vi "PoseInDefenseArea.vi"(5 "theta":dbl, 7 "Recuo":dbl=130.0, 8 "geometry":T1, 9 "Ball":dbl[](array[numeric]), 10 "Field defense":dbl[](array[numeric]), 11 "Events.Ball out":bool) -> (3 "Array":dbl[](array[numeric]))   [LabVIEW 2016]
uses:
  Core/Field Size.ctl
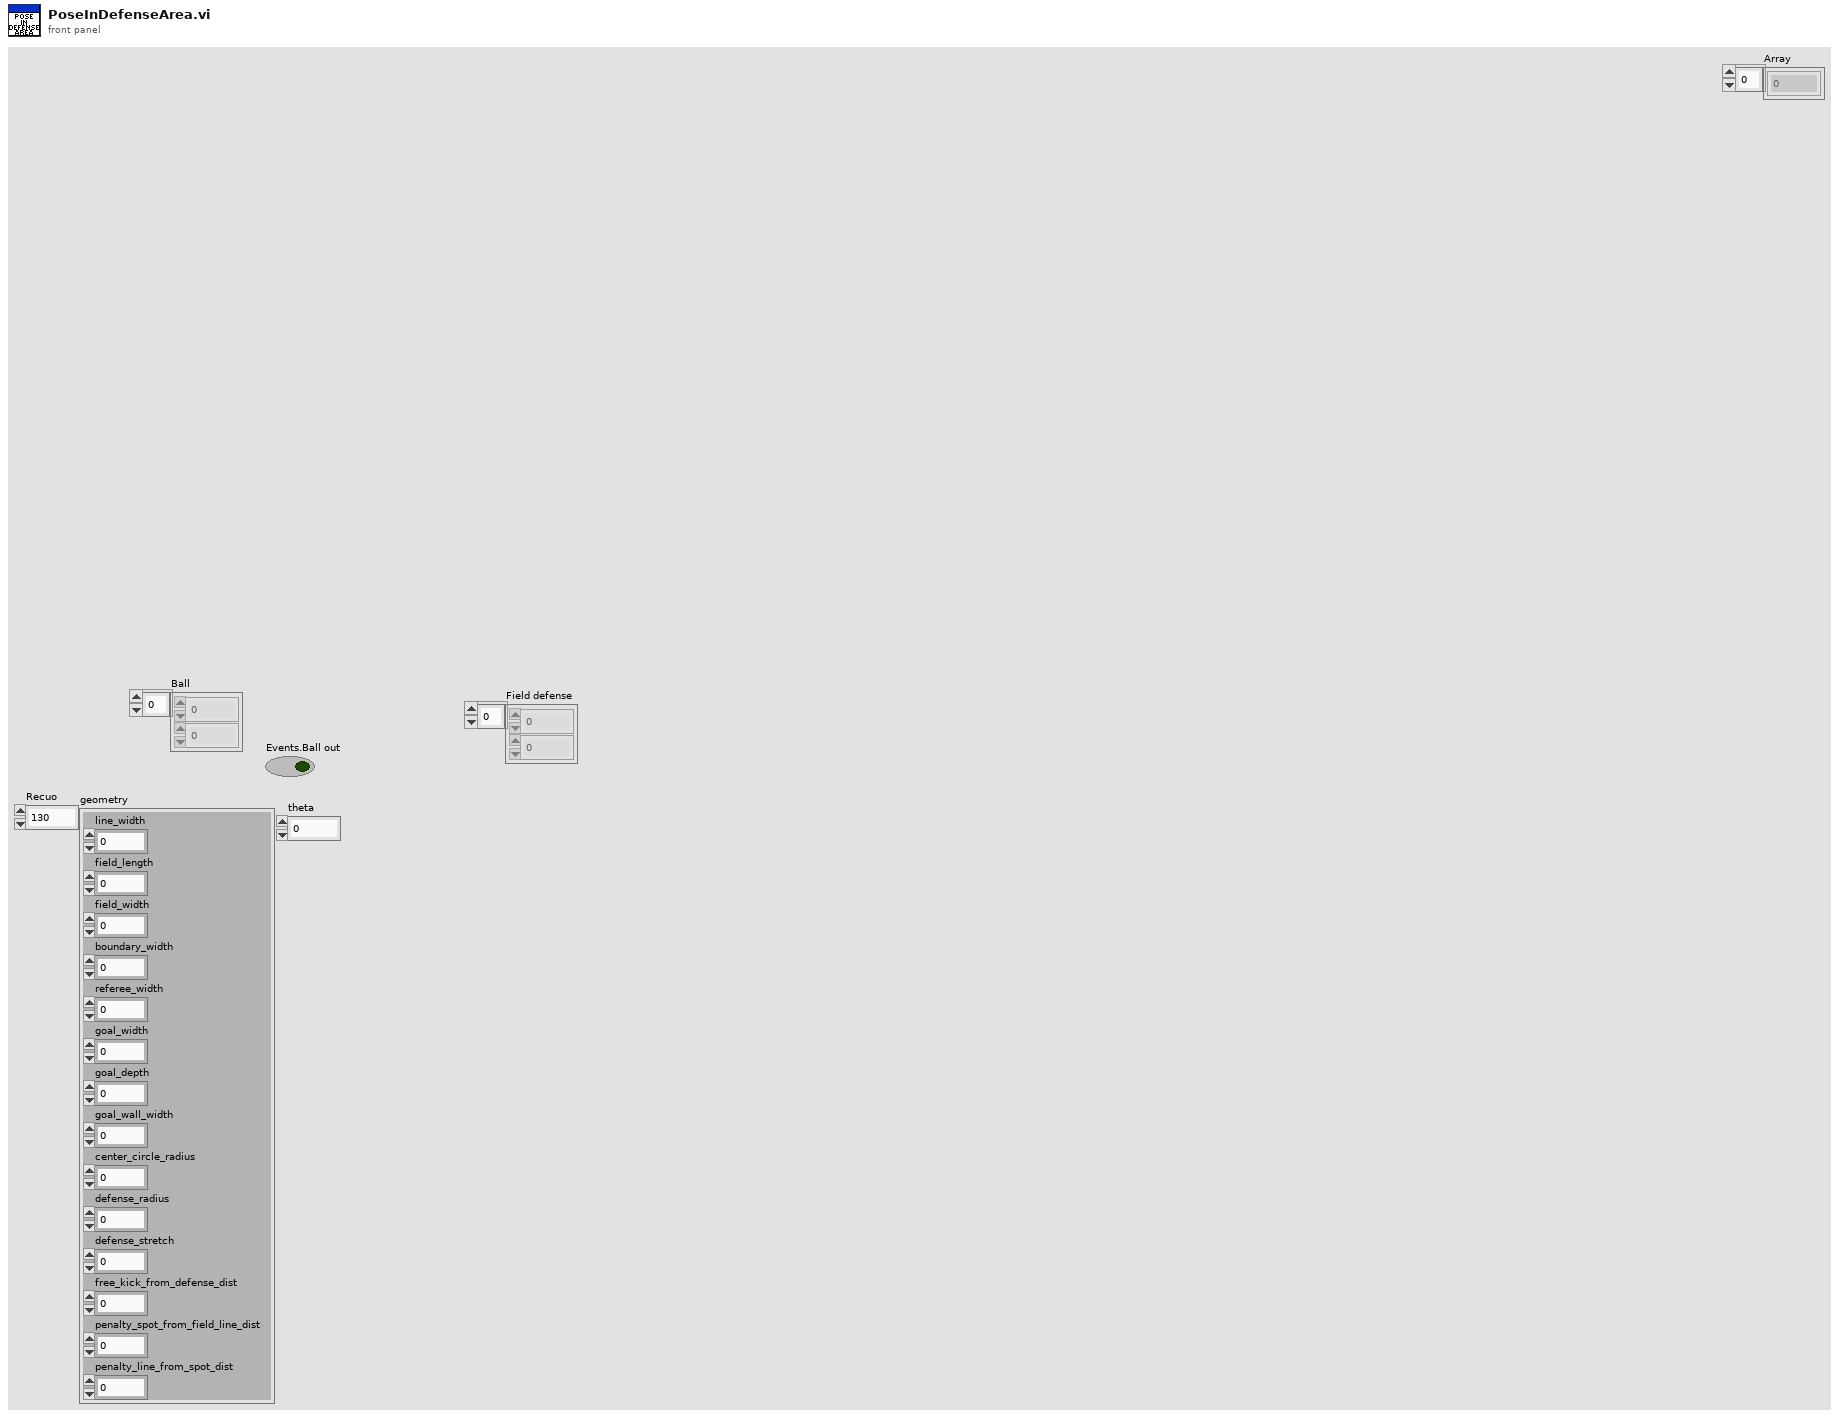
[diagram p1: front panel]
types:
  T1 = typedef "Field Size.ctl" = cluster{"line_width":u32, "field_length":u32, "field_width":u32, "boundary_width":u32, "referee_width":u32, "goal_width":u32, "goal_depth":u32, "goal_wall_width":u32, "center_circle_radius":u32, "defense_radius":u32, "defense_stretch":u32, "free_kick_from_defense_dist":u32, "penalty_spot_from_field_line_dist":u32, "penalty_line_from_spot_dist":u32}
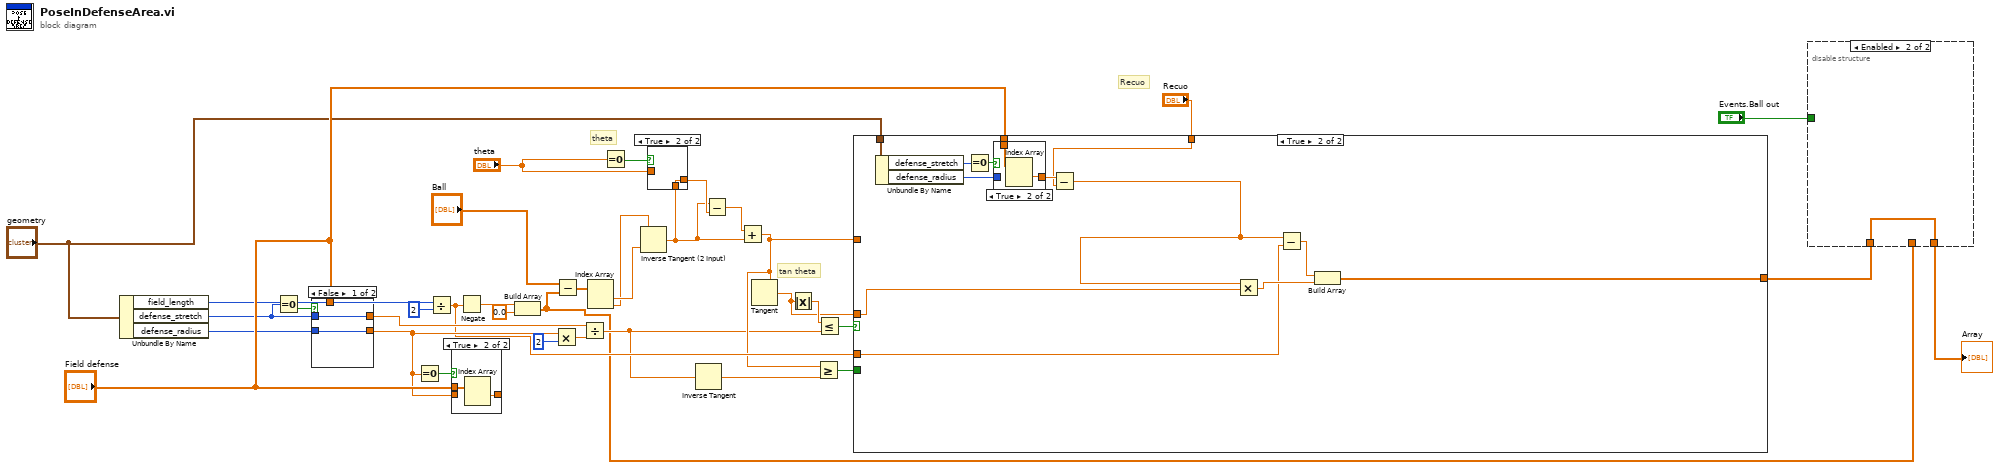
[diagram p0: block diagram]
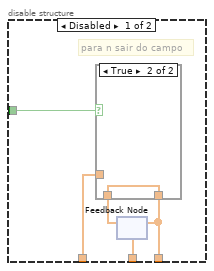
[diagram p2: hidden frame]
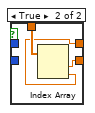
[diagram p5: hidden frame]
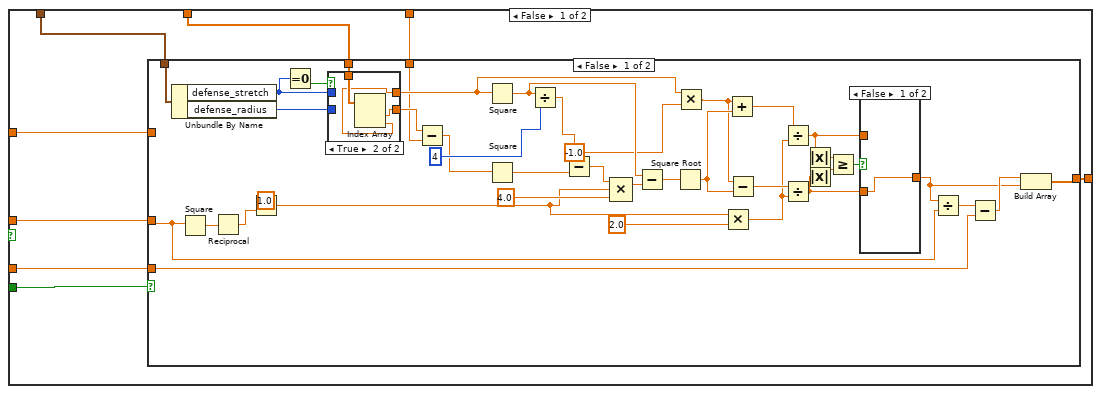
[diagram p6: hidden frame]
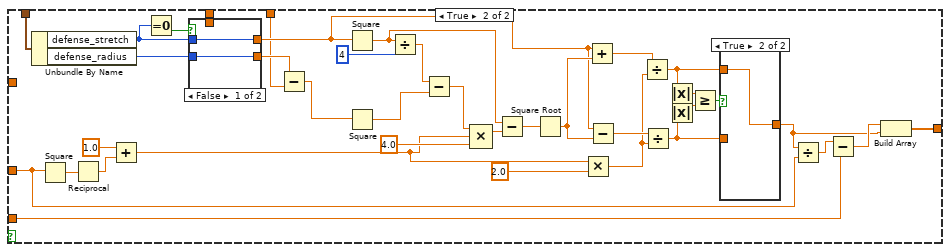
[diagram p9: hidden frame]
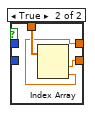
[diagram p10: hidden frame]
diagram:
  # "Recuo"
  # "tan theta"
  # "theta"
  n1 = Unbundle By Name("geometry") -> ("field_length"=w15:u32, "defense_stretch"=w32:u32, "defense_radius"=w31:u32)
  n2 = Equal To 0?(x=w32) -> (x = 0?=w30:bool)
  n3 = case shown="False" w30 {
    tunnel: w32 -> [w38 _]
    tunnel: [w38 w40] -> w34
    tunnel: [w37 w39] -> w33
    tunnel: w31 -> [w37 _]
    tunnel: "Field defense" -> [_ w41]
    frame False {
    }
    frame True {
      n4 = Index Array(array=w41) -> (element #1=w39:dbl, element #2=w40:dbl)  [unwired: 2 in]
    }
  }
  n5 = Equal To 0?(x=w33) -> (x = 0?=w14:bool)
  n6 = Divide(x=w15, y=u32 2) -> (x/y=w27:dbl)
  n7 = case shown="True" w14 {
    tunnel: [w42 w43] -> _
    tunnel: w33 -> [w42 _]
    tunnel: "Field defense" -> [_ w44]
    frame False {
    }
    frame True {
      n8 = Index Array(array=w44) -> (element #2=w43:dbl)  [unwired: 2 in, 1 out]
    }
  }
  n9 = Negate(x=w27) -> (-x=w17:dbl)
  n10 = Build Array(w17, 0.0 ("element")) -> (w2:dbl[])
  n11 = Multiply(x=w33, y=u32 2) -> (x*y=w21:dbl)
  n12 = Subtract(x="Ball", y=w2) -> (x-y=w19:dbl[])
  n13 = Divide(x=w34, y=w21) -> (x/y=w4:dbl)
  n14 = Index Array(array=w19) -> (element #1=w26:dbl, element #2=w25:dbl)  [unwired: 2 in]
  n15 = Equal To 0?(x="theta") -> (x = 0?=w8:bool)
  n16 = Inverse Tangent (2 Input)(1:w26, 2:w25) -> (0:w6:dbl)
  n17 = case shown="True" w8 {
    tunnel: [w45 w46] -> w9
    tunnel: "theta" -> [w45 _]
    tunnel: w6 -> [_ w46]
    frame False {
    }
    frame True {
    }
  }
  n18 = Inverse Tangent(1:w4) -> (0:w3:dbl)
  n19 = Subtract(x=w6, y=w9) -> (x-y=w10:dbl)
  n20 = Add(x=w10, y=w6) -> (x+y=w5:dbl)
  n21 = Tangent(1:w5) -> (0:w11:dbl)
  n22 = Absolute Value(x=w11) -> (abs(x)=w20:dbl)
  n23 = Greater Or Equal?(x=w5, y=w3) -> (x >= y?=w24:bool)
  n24 = Less Or Equal?(x=w20, y=w4) -> (x <= y?=w23:bool)
  n25 = case shown="True" w23 {
    tunnel: w5 -> [w49 _]
    tunnel: "geometry" -> [w53 w157]
    tunnel: [w51 w155] -> w28
    tunnel: w24 -> [w54 _]
    tunnel: w11 -> [w52 w152]
    tunnel: w27 -> [w50 w153]
    tunnel: "Field defense" -> [w48 w146]
    tunnel: "Recuo" -> [w47 w145]
    frame False {
      n26 = case shown="False" w54 {
        tunnel: w53 -> [w76 w137]
        tunnel: w52 -> [w75 w119]
        tunnel: [w74 w118] -> w51
        tunnel: w50 -> [w70 w116]
        tunnel: w49 -> [_ _]
        tunnel: w48 -> [w64 w107]
        tunnel: w47 -> [w55 w101]
        frame False {
          n27 = Unbundle By Name(w76) -> ("defense_stretch"=w61:u32, "defense_radius"=w65:u32)
          n28 = Square(x=w75) -> (x^2=w93:dbl)
          n29 = Reciprocal(x=w93) -> (1/x=w92:dbl)
          n30 = Add(x=1.0, y=w92) -> (x+y=w79:dbl)
          n31 = Equal To 0?(x=w61) -> (x = 0?=w66:bool)
          n32 = case shown="True" w66 {
            tunnel: w61 -> [w95 _]
            tunnel: [w95 w97] -> w63
            tunnel: [w94 w96] -> w62
            tunnel: w65 -> [w94 _]
            tunnel: w64 -> [_ w98]
            frame False {
            }
            frame True {
              n33 = Index Array(array=w98) -> (element #1=w96:dbl, element #2=w97:dbl)  [unwired: 2 in]
            }
          }
          n34 = Subtract(x=w62, y=w55) -> (x-y=w67:dbl)
          n35 = Square(x=w63) -> (x^2=w87:dbl)
          n36 = Square(x=w67) -> (x^2=w88:dbl)
          n37 = Divide(x=w87, y=u32 4) -> (x/y=w89:dbl)
          n38 = Subtract(x=w89, y=w88) -> (x-y=w85:dbl)
          n39 = Compound Arithmetic op=MULTIPLY(w85, w79, 4.0 ("value")) -> (w86:dbl)
          n40 = Subtract(x=w87, y=w86) -> (x-y=w83:dbl)
          n41 = Square Root(x=w83) -> (sqrt(x)=w82:dbl)
          n42 = Multiply(x=w63, y=-1.0) -> (x*y=w73:dbl)
          n43 = Multiply(x=w79, y=2.0) -> (x*y=w77:dbl)
          n44 = Add(x=w73, y=w82) -> (x+y=w81:dbl)
          n45 = Subtract(x=w73, y=w82) -> (x-y=w80:dbl)
          n46 = Divide(x=w81, y=w77) -> (x/y=w58:dbl)
          n47 = Divide(x=w80, y=w77) -> (x/y=w56:dbl)
          n48 = Absolute Value(x=w58) -> (abs(x)=w59:dbl)
          n49 = Absolute Value(x=w56) -> (abs(x)=w57:dbl)
          n50 = Greater Or Equal?(x=w59, y=w57) -> (x >= y?=w60:bool)
          n51 = case shown="False" w60 {
            tunnel: w56 -> [w99 _]
            tunnel: [w99 w100] -> w68
            tunnel: w58 -> [_ w100]
            frame False {
            }
            frame True {
            }
          }
          n52 = Divide(x=w68, y=w75) -> (x/y=w69:dbl)
          n53 = Subtract(x=w69, y=w70) -> (x-y=w71:dbl)
          n54 = Build Array(w71, w68) -> (w74:dbl[])
        }
        frame True {
          n55 = Unbundle By Name(w137) -> ("defense_stretch"=w109:u32, "defense_radius"=w110:u32)
          n56 = Square(x=w119) -> (x^2=w136:dbl)
          n57 = Reciprocal(x=w136) -> (1/x=w135:dbl)
          n58 = Add(x=1.0, y=w135) -> (x+y=w122:dbl)
          n59 = Equal To 0?(x=w109) -> (x = 0?=w108:bool)
          n60 = case shown="False" w108 {
            tunnel: w109 -> [w139 _]
            tunnel: [w139 w141] -> w112
            tunnel: [w138 w140] -> w111
            tunnel: w110 -> [w138 _]
            tunnel: w107 -> [_ w142]
            frame False {
            }
            frame True {
              n61 = Index Array(array=w142) -> (element #1=w140:dbl, element #2=w141:dbl)  [unwired: 2 in]
            }
          }
          n62 = Subtract(x=w111, y=w101) -> (x-y=w113:dbl)
          n63 = Square(x=w112) -> (x^2=w130:dbl)
          n64 = Square(x=w113) -> (x^2=w131:dbl)
          n65 = Divide(x=w130, y=u32 4) -> (x/y=w132:dbl)
          n66 = Subtract(x=w132, y=w131) -> (x-y=w128:dbl)
          n67 = Compound Arithmetic op=MULTIPLY(w128, w122, 4.0 ("value")) -> (w129:dbl)
          n68 = Subtract(x=w130, y=w129) -> (x-y=w126:dbl)
          n69 = Square Root(x=w126) -> (sqrt(x)=w125:dbl)
          n70 = Multiply(x=w122, y=2.0) -> (x*y=w120:dbl)
          n71 = Add(x=w112, y=w125) -> (x+y=w124:dbl)
          n72 = Subtract(x=w112, y=w125) -> (x-y=w123:dbl)
          n73 = Divide(x=w124, y=w120) -> (x/y=w104:dbl)
          n74 = Divide(x=w123, y=w120) -> (x/y=w103:dbl)
          n75 = Absolute Value(x=w104) -> (abs(x)=w102:dbl)
          n76 = Absolute Value(x=w103) -> (abs(x)=w106:dbl)
          n77 = Greater Or Equal?(x=w102, y=w106) -> (x >= y?=w105:bool)
          n78 = case shown="True" w105 {
            tunnel: w103 -> [w143 _]
            tunnel: [w143 w144] -> w114
            tunnel: w104 -> [_ w144]
            frame False {
            }
            frame True {
            }
          }
          n79 = Divide(x=w114, y=w119) -> (x/y=w115:dbl)
          n80 = Subtract(x=w115, y=w116) -> (x-y=w117:dbl)
          n81 = Build Array(w117, w114) -> (w118:dbl[])
        }
      }
    }
    frame True {
      n82 = Unbundle By Name(w157) -> ("defense_stretch"=w147:u32, "defense_radius"=w149:u32)
      n83 = Equal To 0?(x=w147) -> (x = 0?=w148:bool)
      n84 = case shown="True" w148 {
        tunnel: [w158 w159] -> w150
        tunnel: w149 -> [w158 _]
        tunnel: w146 -> [_ w160]
        frame False {
        }
        frame True {
          n85 = Index Array(array=w160) -> (element #1=w159:dbl)  [unwired: 2 in, 1 out]
        }
      }
      n86 = Subtract(x=w150, y=w145) -> (x-y=w151:dbl)
      n87 = Multiply(x=w151, y=w152) -> (x*y=w156:dbl)
      n88 = Subtract(x=w151, y=w153) -> (x-y=w154:dbl)
      n89 = Build Array(w154, w156) -> (w155:dbl[])
    }
  }
  n90 = disable-structure shown="Enabled" {
    disable-tunnel: [w165 w168] -> w29
    disable-tunnel: w28 -> [w164 w168]
    disable-tunnel: w2 -> [w162 _]
    disable-tunnel: "Events.Ball out" -> [w161 _]
    frame Disabled {
      # "para n sair do campo"
      n91 = feedback #1(w162) -> (w163:dbl[])
      n92 = case shown="True" w161 {
        tunnel: w163 -> [_ w167]
        tunnel: w164 -> [w166 _]
        tunnel: [w166 w167] -> w165
        frame False {
        }
        frame True {
        }
      }
      n93 = feedback-in #1(w165) -> ()
    }
    frame Enabled {
    }
  }
  "Array" <- w29
